vi "NewReportPage_SFP_86To85.vi"(9 "Scratchpad Diagram (Contains XNode)":refnum<vi>, 10 "XRef (Scratchpad Diagram)":refnum<vi>, 11 "XRef (Original Diagram)":refnum<vi>) -> (1 "Custom Label":string, 2 "Custom Warning To Issue":string, 3 "Action":T1)   [LabVIEW 2020]
uses:
  <vilib>/XSFPSupport/SFPReplaceAction.ctl
  <vilib>/XSFPSupport/NI_XSFPSupport.lvlib
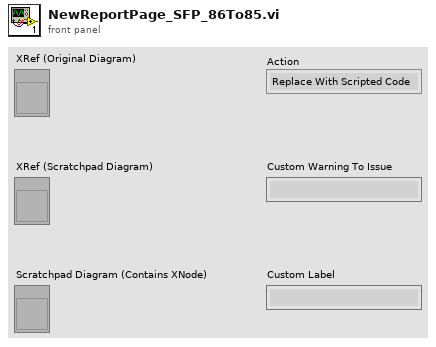
[diagram p1: front panel]
types:
  T1 = typedef "NI_XSFPSupport.lvlib/SFPReplaceAction.ctl" = enum32{"Replace With Scripted Code", "Replace With Label", "Fail SFP"}
  T2 = typedef "LVPositionTypeDef.ctl" = cluster{"Left":i32, "Top":i32}
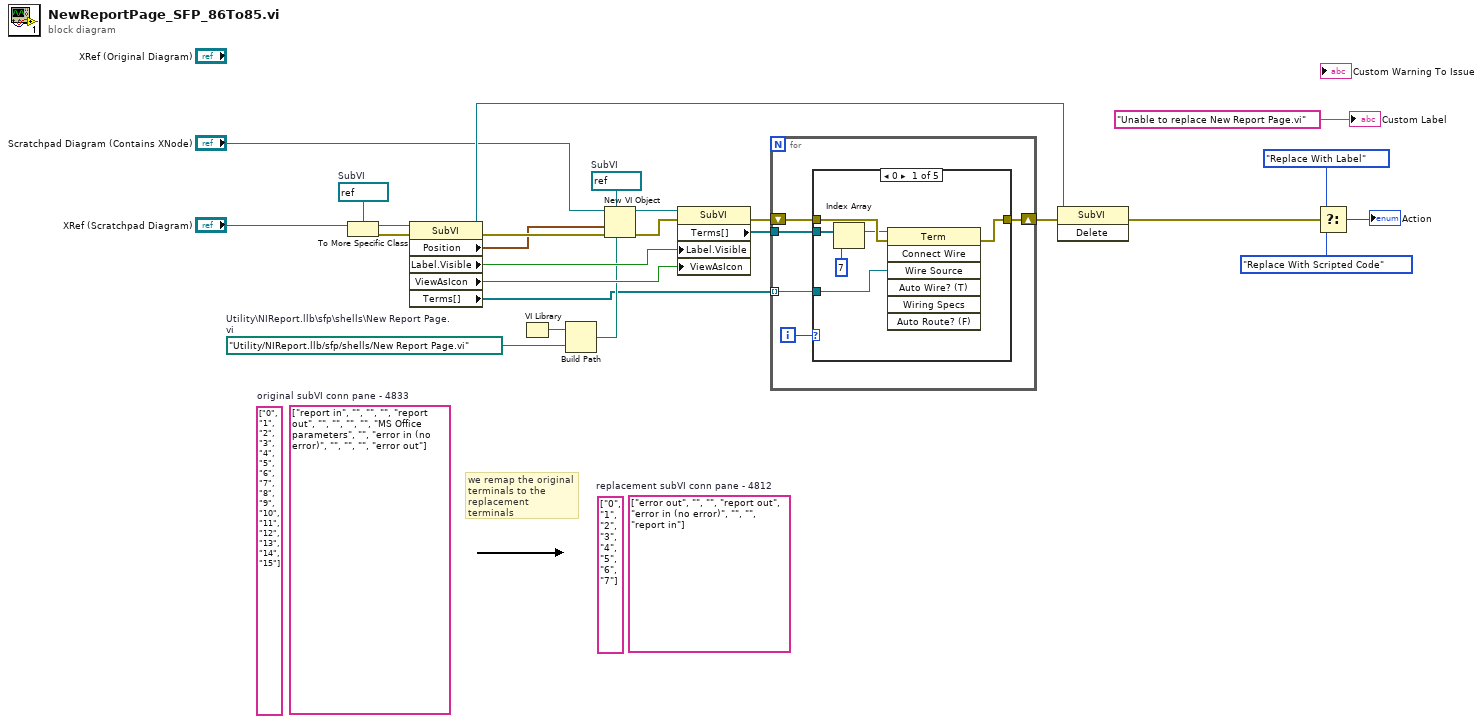
[diagram p0: block diagram]
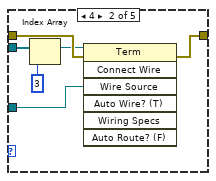
[diagram p2: hidden frame]
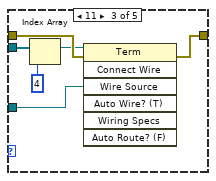
[diagram p3: hidden frame]
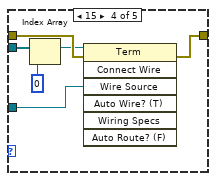
[diagram p4: hidden frame]
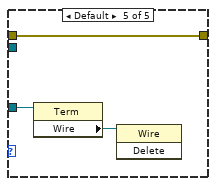
[diagram p5: hidden frame]
diagram:
  (unwired) string[] ["0", "1", "2", "3", "4", "5", "6", "7", "8", "9", "10", "11", "12", "13", "14", "15"]
  (unwired) string[] ["0", "1", "2", "3", "4", "5", "6", "7"]
  (unwired) string[] ["report in", "", "", "", "report out", "", "", "", "", "MS Office parameters", "", "error in (no error)", "", "", "", "error out"]  # original subVI conn pane - 4833
  (unwired) string[] ["error out", "", "", "report out", "error in (no error)", "", "", "report in"]  # replacement subVI conn pane - 4812
  w6 = path "Utility/NIReport.llb/sfp/shells/New Report Page.vi"  # Utility\NIReport.llb\sfp\shells\New Report Page.vi
  w15 = refnum<vi> refnum  # SubVI
  w18 = refnum<vi> refnum  # SubVI
  # "we remap the original terminals to the replacement terminals"
  n1 = To More Specific Class(target class=w18, reference="XRef (Scratchpad Diagram)") -> (specific class reference=w17:refnum<vi>, error out=w25:errorcluster)  [unwired: 1 in]
  n2 = property class="SubVI"(reference=w17, error in=w25) -> (reference out=w5:refnum<vi>, error out=w24:errorcluster, "Position"=w16:T2, "Label.Visible"=w13:bool, "ViewAsIcon"=w12:bool, "Terms[]"=w2:refnum<vi>[])
  n3 = VI Library() -> (path=w7:path)
  n4 = Build Path(base path=w7, name or relative path=w6) -> (appended path=w4:path)
  n5 = New VI Object(vi object class=w15, owner refnum="Scratchpad Diagram (Contains XNode)", position/next to=w16, 6:w4, 8:w24) -> (object refnum=w14:refnum<vi>, 0:w23:errorcluster)  [unwired: 3 out]
  n6 = property class="SubVI"(reference=w14, error in=w23, "Label.Visible"=w13, "ViewAsIcon"=w12) -> (error out=w21:errorcluster, "Terms[]"=w1:refnum<vi>[])  [unwired: 1 out]
  n7 = for {
    tunnel: w1 -> [w28]
    tunnel: w2 -> [w26] mode=indexing
    shift-right: [w29] -> w20
    shift-left: w21 -> [w30]
    i -> [w27]
    n8 = case shown="0" w27 {
      tunnel: w28 -> [w33 w39 w45 w51 _]
      tunnel: w26 -> [w32 w38 w44 w50 w56]
      tunnel: w30 -> [w36 w42 w48 w54 w57]
      tunnel: [w35 w41 w47 w53 w57] -> w29
      frame 0 {
        n9 = Index Array(array=w33, index=7) -> (element=w31:refnum<vi>)
        n10 = invoke class="Term" method="Connect Wire"(reference=w31, error in=w36, "Wire Source"=w32) -> (error out=w35:errorcluster)  [unwired: 4 in, 6 out]
      }
      frame 4 {
        n11 = Index Array(array=w39, index=3) -> (element=w37:refnum<vi>)
        n12 = invoke class="Term" method="Connect Wire"(reference=w37, error in=w42, "Wire Source"=w38) -> (error out=w41:errorcluster)  [unwired: 4 in, 6 out]
      }
      frame 11 {
        n13 = Index Array(array=w45, index=4) -> (element=w43:refnum<vi>)
        n14 = invoke class="Term" method="Connect Wire"(reference=w43, error in=w48, "Wire Source"=w44) -> (error out=w47:errorcluster)  [unwired: 4 in, 6 out]
      }
      frame 15 {
        n15 = Index Array(array=w51, index=0) -> (element=w49:refnum<vi>)
        n16 = invoke class="Term" method="Connect Wire"(reference=w49, error in=w54, "Wire Source"=w50) -> (error out=w53:errorcluster)  [unwired: 4 in, 6 out]
      }
      frame Default {
        n17 = property class="Term"(reference=w56) -> ("Wire"=w55:refnum<vi>)  [unwired: 1 in, 2 out]
        n18 = invoke class="Wire" method="Delete"(reference=w55) -> ()  [unwired: 2 in, 3 out]
      }
    }
  }
  n19 = invoke class="SubVI" method="Delete"(reference=w5, error in=w20) -> (error out=w22:errorcluster)  [unwired: 1 in, 2 out]
  n20 = Select(t=SFPReplaceAction."Replace With Label" ("Action"), s=w22, f=SFPReplaceAction."Replace With Scripted Code" ("Action")) -> (s? t:f=→"Action":T1)
  "Custom Label" <- "Unable to replace New Report Page.vi" ("Custom Label")
